vi "TwoBallAuton2.vi"() -> ()   [LabVIEW 2013]
uses:
  Events.vi
  AutonVars.vi
panel:
  out "WaitTime":dbl=3000.0
  out "TimeDriveFoward":dbl=2000.0
  out "Backward Speed":dbl=-0.68
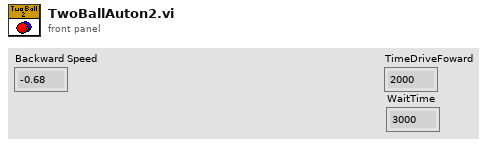
[diagram p1: front panel]
types:
  T1 = cluster{"Translate":dbl, "Y-Axis (Backward Speed)":dbl, "Rotate":dbl, "Tank right side":dbl, "axis 5":dbl, "axis 6":dbl, "Use gyro":bool, "Exponential\ndrive":bool, "Ring light":bool, "PID rotation":bool, "PID Gain":dbl}
  T2 = typedef "Eventgrab.ctl" = cluster{"Grab":bool, "GroundPass":bool, "Test Aqaure":dbl, "Shoulder up or down?":bool, "Auton drag":bool}
  T3 = cluster{"Reloading?":bool, "Throw":bool, "Ready?":bool, "Truss throw":bool, "Power is high?":bool, "Automatic relaod?":bool, "Manuall servo":bool}
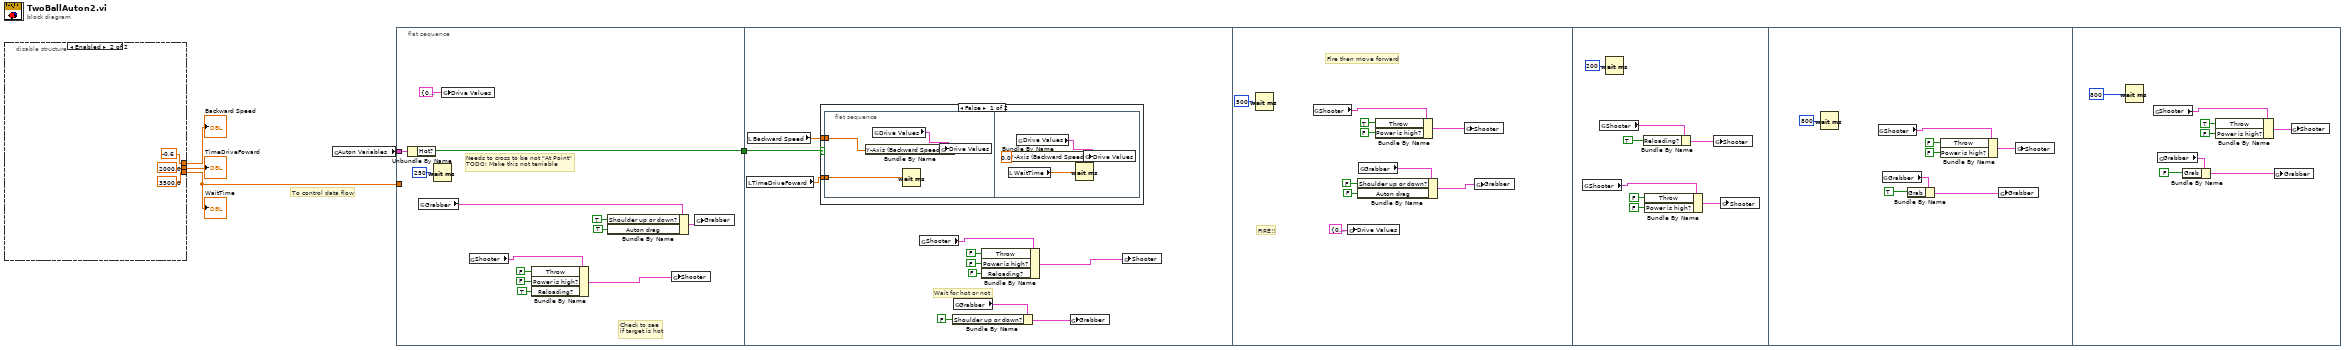
[diagram p0: block diagram]
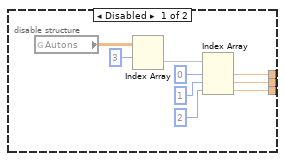
[diagram p2: hidden frame]
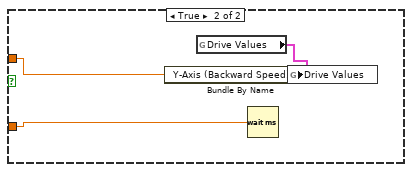
[diagram p3: hidden frame]
diagram:
  # "To control data flow"
  n1 = disable-structure shown="Enabled" {
    disable-tunnel: [w11 -0.6 ("Backward Speed")] -> w3
    disable-tunnel: [w10 2000.0 ("TimeDriveFoward")] -> w2
    disable-tunnel: [w6 3500.0 ("WaitTime")] -> w1
    frame Disabled {
      n2 = global read "AutonVars.vi" "Autons"() -> (w9:dbl[][])
      n3 = Index Array(array=w9, index (row)=3) -> (element=w7:dbl[])  [unwired: 1 in]
      n4 = Index Array(array=w7, index #1=0 ("index"), index #2=1 ("index"), index #3=2 ("index")) -> (element #1=w11:dbl, element #2=w10:dbl, element #3=w6:dbl)
    }
    frame Enabled {
    }
  }
  "Backward Speed" <- w3
  "TimeDriveFoward" <- w2
  "WaitTime" <- w1
  n5 = global read "Events.vi" "Auton Variables"() -> (w4:cluster{"Hot?":bool, "WhichAuton":string})
  n6 = flat-sequence {
    tunnel: [w30] -> w5
    tunnel: w4 -> [w28]
    tunnel: w1 -> [_]
    tunnel: w5 -> [w38]
    frame #0 {
      # "Needs to cross to be not \"At Point\"\nTODO: Make this not terriable"
      # "Check to see\nif target is hot"
      n7 = Unbundle By Name(w28) -> ("Hot?"=w30:bool)
      n8 = global read "Events.vi" "Grabber"() -> (w26:T2)
      n9 = Wait (ms)(milliseconds to wait=u32 250) -> ()  [unwired: 1 out]
      n10 = global write "Events.vi" "Drive Values"(T1 {"Translate"=0.0, "Y-Axis (Backward Speed)"=0.0, "Rotate"=0.0, "Tank right side"=0.0, "axis 5"=0.0, "axis 6"=0.0, "Use gyro"=FALSE, "Exponential\ndrive"=TRUE, "Ring light"=FALSE, "PID rotation"=FALSE, "PID Gain"=0.0} ("Drive Values")) -> ()
      n11 = global read "Events.vi" "Shooter"() -> (w24:T3)
      n12 = Bundle By Name(cluster=w24, "Throw"=FALSE, "Power is high?"=FALSE, "Reloading?"=TRUE) -> (w23:T3)
      n13 = Bundle By Name(cluster=w26, "Shoulder up or down?"=TRUE, "Auton drag"=TRUE) -> (w25:T2)
      n14 = global write "Events.vi" "Shooter"(w23) -> ()
      n15 = global write "Events.vi" "Grabber"(w25) -> ()
    }
    frame #1 {
      # "Wait for hot or not"
      n16 = local read "TimeDriveFoward"() -> (w31:dbl)
      n17 = local read "Backward Speed"() -> (w32:dbl)
      n18 = case shown="False" w38 {
        tunnel: w32 -> [w43 w53]
        tunnel: w31 -> [w42 w52]
        frame False {
          n19 = flat-sequence {
            tunnel: w43 -> [w45]
            tunnel: w42 -> [w44]
            frame #0 {
              n20 = global read "Events.vi" "Drive Values"() -> (w46:T1)
              n21 = Bundle By Name(cluster=w46, "Y-Axis (Backward Speed)"=w45) -> (w47:T1)
              n22 = Wait (ms)(milliseconds to wait=w44) -> ()  [unwired: 1 out]
              n23 = global write "Events.vi" "Drive Values"(w47) -> ()
            }
            frame #1 {
              n24 = local read "WaitTime"() -> (w48:dbl)
              n25 = global read "Events.vi" "Drive Values"() -> (w50:T1)
              n26 = Bundle By Name(cluster=w50, "Y-Axis (Backward Speed)"=0.0 ("Forward Speed")) -> (w51:T1)
              n27 = Wait (ms)(milliseconds to wait=w48) -> ()  [unwired: 1 out]
              n28 = global write "Events.vi" "Drive Values"(w51) -> ()
            }
          }
        }
        frame True {
          n29 = global read "Events.vi" "Drive Values"() -> (w54:T1)
          n30 = Bundle By Name(cluster=w54, "Y-Axis (Backward Speed)"=w53) -> (w55:T1)
          n31 = Wait (ms)(milliseconds to wait=w52) -> ()  [unwired: 1 out]
          n32 = global write "Events.vi" "Drive Values"(w55) -> ()
        }
      }
      n33 = global read "Events.vi" "Shooter"() -> (w37:T3)
      n34 = global read "Events.vi" "Grabber"() -> (w40:T2)
      n35 = Bundle By Name(cluster=w40, "Shoulder up or down?"=FALSE) -> (w41:T2)
      n36 = Bundle By Name(cluster=w37, "Throw"=FALSE, "Power is high?"=FALSE, "Reloading?"=FALSE) -> (w36:T3)
      n37 = global write "Events.vi" "Grabber"(w41) -> ()
      n38 = global write "Events.vi" "Shooter"(w36) -> ()
    }
    frame #2 {
      # "FIRE!!"
      # "Fire then move forward"
      n39 = Wait (ms)(milliseconds to wait=u32 500) -> ()  [unwired: 1 out]
      n40 = global read "Events.vi" "Shooter"() -> (w65:T3)
      n41 = global write "Events.vi" "Drive Values"(T1 {"Translate"=0.0, "Y-Axis (Backward Speed)"=0.0, "Rotate"=0.0, "Tank right side"=0.0, "axis 5"=0.0, "axis 6"=0.0, "Use gyro"=FALSE, "Exponential\ndrive"=TRUE, "Ring light"=FALSE, "PID rotation"=FALSE, "PID Gain"=0.0} ("Drive Values")) -> ()
      n42 = global read "Events.vi" "Grabber"() -> (w58:T2)
      n43 = Bundle By Name(cluster=w58, "Shoulder up or down?"=FALSE, "Auton drag"=FALSE) -> (w60:T2)
      n44 = Bundle By Name(cluster=w65, "Throw"=TRUE, "Power is high?"=FALSE) -> (w64:T3)
      n45 = global write "Events.vi" "Shooter"(w64) -> ()
      n46 = global write "Events.vi" "Grabber"(w60) -> ()
    }
    frame #3 {
      n47 = global read "Events.vi" "Shooter"() -> (w69:T3)
      n48 = global read "Events.vi" "Shooter"() -> (w73:T3)
      n49 = Wait (ms)(milliseconds to wait=u32 200) -> ()  [unwired: 1 out]
      n50 = Bundle By Name(cluster=w73, "Reloading?"=TRUE ("Throw")) -> (w72:T3)
      n51 = Bundle By Name(cluster=w69, "Throw"=FALSE, "Power is high?"=FALSE) -> (w68:T3)
      n52 = global write "Events.vi" "Shooter"(w72) -> ()
      n53 = global write "Events.vi" "Shooter"(w68) -> ()
    }
    frame #4 {
      n54 = Wait (ms)(milliseconds to wait=u32 800) -> ()  [unwired: 1 out]
      n55 = global read "Events.vi" "Shooter"() -> (w81:T3)
      n56 = global read "Events.vi" "Grabber"() -> (w74:T2)
      n57 = Bundle By Name(cluster=w74, "Grab"=TRUE ("Shoulder up or down?")) -> (w76:T2)
      n58 = Bundle By Name(cluster=w81, "Throw"=FALSE, "Power is high?"=FALSE) -> (w80:T3)
      n59 = global write "Events.vi" "Grabber"(w76) -> ()
      n60 = global write "Events.vi" "Shooter"(w80) -> ()
    }
    frame #5 {
      n61 = Wait (ms)(milliseconds to wait=u32 800) -> ()  [unwired: 1 out]
      n62 = global read "Events.vi" "Shooter"() -> (w89:T3)
      n63 = global read "Events.vi" "Grabber"() -> (w82:T2)
      n64 = Bundle By Name(cluster=w82, "Grab"=FALSE ("Shoulder up or down?")) -> (w84:T2)
      n65 = Bundle By Name(cluster=w89, "Throw"=TRUE, "Power is high?"=FALSE) -> (w88:T3)
      n66 = global write "Events.vi" "Grabber"(w84) -> ()
      n67 = global write "Events.vi" "Shooter"(w88) -> ()
    }
  }
